vi "SingleChannelDisplay.vi"(2 "Channel Setting":T1 {"Meas Range" items=["-0.1 V~+0.1 V"=0.1, "-0.2 V~0.2 V"=0.2, "-0.5 V~+0.5 V"=0.5, "-1 V~+1 V"=1.0, "-2 V~+2 V"=2.0, "-5 V~+5 V"=5.0, "-10 V~+10 V"=10.0]; "Vertical\nPosition (Div)" min=-5.0 max=5.0 step=0.01 scale=-5.0..5.0 scale format="%.2f"; "Scale\n  Volts/Div" scale=0.01..20.0}, 3 "Data In":waveform(dbl) caption="Data_In") -> (0 "Data_for_Display":waveform(dbl), 1 "Data_for_measure_out":waveform(dbl))   [LabVIEW 2012]
uses:
  <vilib>/Analysis/NI_AALPro.lvlib
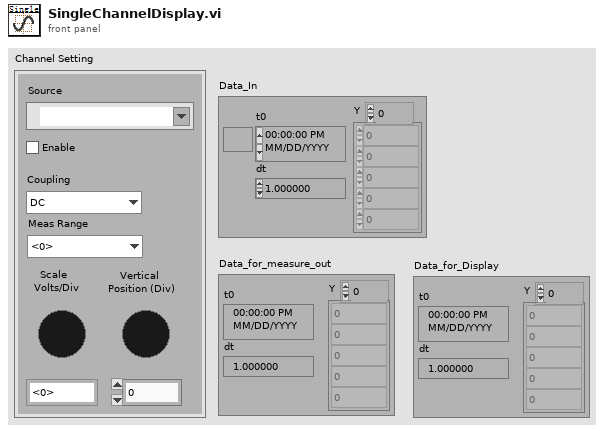
[diagram p1: front panel]
types:
  T1 = cluster{"physical channels":tag, "Enable":bool, "Coupling":enum16{"DC", "AC"}, "    Scale\n  Volts/Div  ":dbl, "    Vertical\nPosition (Div)":dbl, "Meas Range":dbl}
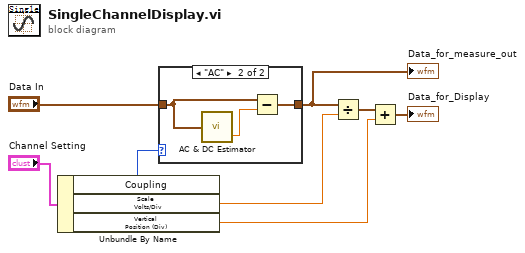
[diagram p0: block diagram]
diagram:
  n1 = Unbundle By Name("Channel Setting") -> ("Coupling"=w6:enum16{"DC", "AC"}, "Scale\n  Volts/Div"=w4:dbl, "Vertical\nPosition (Div)"=w3:dbl)
  n2 = case shown="\"AC\"" w6 {
    tunnel: "Data In" -> [w9 w11]
    tunnel: [w9 w10] -> w2
    frame "DC", Default {
    }
    frame "AC" {
      n3 = call <vilib>:"AC & DC Estimator.vi"("Signal (V)"=w11) -> ("DC estimate (V)"=w12:dbl)  [unwired: 1 out]
      n4 = Subtract(x=w11, y=w12) -> (x-y=w10:waveform(dbl))
    }
  }
  "Data_for_measure_out" <- w2
  n5 = Divide(x=w2, y=w4) -> (x/y=w8:waveform(dbl))
  n6 = Add(x=w8, y=w3) -> (x+y=→"Data_for_Display":waveform(dbl))
